vi "Parameters.vi"() -> ()   [LabVIEW 2019]
panel:
  in  "GlobalString":string
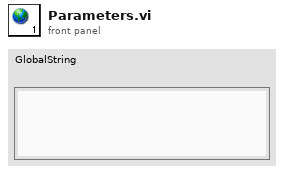
[diagram p1: front panel]
diagram:
